vi "当前时间解析-8.6.vi"(5 "需要秒？(T)":bool=TRUE) -> (10 "日期字符串":string, 11 "名称格式时间":string, 12 "时间字符串":string, 13 "时间":string, 14 "年":u8, 15 "月":u8, 16 "日":u8, 17 "时":u8, 18 "分":u8, 19 "秒":u8)   [LabVIEW 2013]
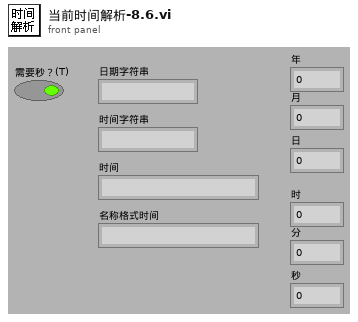
[diagram p1: front panel]
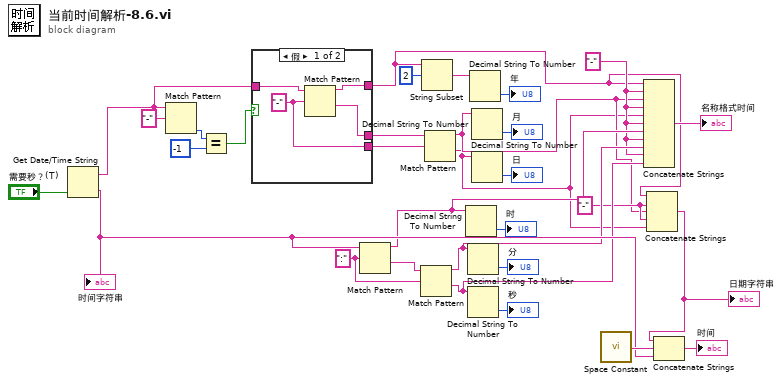
[diagram p0: block diagram]
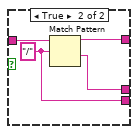
[diagram p2: hidden frame]
diagram:
  w5 = "-"
  w13 = "-"
  w22 = ":" ("正则表达式")
  n1 = Get Date/Time String(want seconds? (F)="需要秒？(T)") -> (date string=w8:string, time string=w19:string)  [unwired: 2 out]
  "时间字符串" <- w19
  n2 = Match Pattern(string=w8, regular expression="-" ("正则表达式")) -> (offset past match=w11:i32)  [unwired: 4 out]
  n3 = Equal?(x=w11, y=-1) -> (x = y?=w9:bool)
  n4 = case shown="假" w9 {
    tunnel: w8 -> [w34 w39]
    tunnel: [w35 w38] -> w4
    tunnel: [w33 w37] -> w7
    tunnel: [w32 w36] -> w6
    frame False {
      w32 = "-" ("正则表达式")
      n5 = Match Pattern(string=w34, regular expression=w32) -> (before substring=w35:string, after substring=w33:string)  [unwired: 3 out]
    }
    frame True {
      w36 = "/" ("正则表达式")
      n6 = Match Pattern(string=w39, regular expression=w36) -> (before substring=w38:string, after substring=w37:string)  [unwired: 3 out]
    }
  }
  n7 = Match Pattern(string=w19, regular expression=w22) -> (before substring=w17:string, after substring=w23:string)  [unwired: 3 out]
  n8 = Match Pattern(string=w23, regular expression=w22) -> (before substring=w16:string, after substring=w15:string)  [unwired: 3 out]
  n9 = String Subset(string=w4, offset (0)=2 ("偏移量(0)")) -> (substring=w12:string)  [unwired: 1 out]
  n10 = Match Pattern(string=w7, regular expression=w6) -> (before substring=w3:string, after substring=w2:string)  [unwired: 3 out]
  n11 = Decimal String To Number(string=w17) -> (number=→"时":i32)  [unwired: 3 out]
  n12 = Decimal String To Number(string=w16) -> (number=→"分":i32)  [unwired: 3 out]
  n13 = Decimal String To Number(string=w15) -> (number=→"秒":i32)  [unwired: 3 out]
  n14 = Decimal String To Number(string=w12) -> (number=→"年":i32)  [unwired: 3 out]
  n15 = Decimal String To Number(string=w3) -> (number=→"月":i32)  [unwired: 3 out]
  n16 = Decimal String To Number(string=w2) -> (number=→"日":i32)  [unwired: 3 out]
  n17 = call <vilib>:"Space Constant.vi"() -> ("String"=w20:string)
  n18 = Concatenate Strings(w4, w13, w3, w13, w2, w13, w17, w13, w16, w13, w15) -> (→"名称格式时间":string)
  n19 = Concatenate Strings(w4, w5, w3, w5, w2) -> (w1:string)
  "日期字符串" <- w1
  n20 = Concatenate Strings(w1, w20, w19) -> (→"时间":string)
